vi "Close Hardware.vi"(8 "error in (no error)":errorcluster, 11 "Instrument.VRM in":refnum<class "Instrument.OxfordVRM.lvclass">) -> (0 "error out":errorcluster, 3 "Instrument.VRM out":refnum<class "Instrument.OxfordVRM.lvclass">)   [LabVIEW 2019, in "Instrument.OxfordVRM.lvclass"]
uses:
  Instrument.OxfordVRM.lvclass
  <instrlib>/Mercury iXX/Public/Controls/Mercury Reference.ctl
  <instrlib>/Mercury iXX/Public/Controls/Comms Transport Layer.ctl
  <instrlib>/Mercury iXX/Private/Controls/Query Dynamic Reference.ctl
  Instrument.OxfordVRM.lvclass/Instrument.OxfordVRM.ctl
  <instrlib>/Mercury iXX/Mercury iXX.lvlib
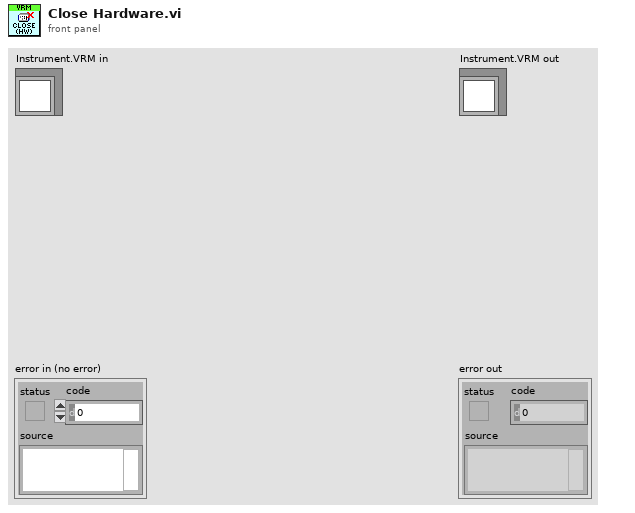
[diagram p1: front panel]
types:
  T1 = typedef "Mercury iXX.lvlib/Mercury Reference.ctl" = cluster{"Comms":refnum<visa-resource-name>, "Device ID":string[], "Comms Layer":T2, "Command":string, "Query reference":T3}
  T2 = typedef "Mercury iXX.lvlib/Comms Transport Layer.ctl" = enum16{"Ethernet TCP/IP", "USB", "ISOBus - RS-232", "GPIB"}
  T3 = typedef "Mercury iXX.lvlib/Query Dynamic Reference.ctl" = refnum<vi>
  T4 = cluster{"Reference":T1, "Devices":cluster{"Temperature":string, "Magnet X":string, "Magnet Y":string, "Magnet Z":string, "PSU 1":string, "PSU 2":string, "PSU 3":string, "PSU 4":string, "PSU 5":string, "PSU 6":string}}
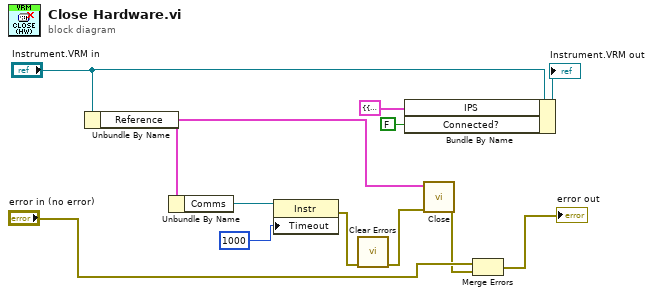
[diagram p0: block diagram]
diagram:
  n1 = Unbundle By Name("Instrument.VRM in") -> ("Reference"=w5:T1)
  n2 = Unbundle By Name(w5) -> ("Comms"=w8:refnum<visa-resource-name>)
  n3 = property class="Instr"(reference=w8, "Timeout"=u32 1000 ("General Settings:Timeout Value")) -> (error out=w6:errorcluster)  [unwired: 1 in, 1 out]
  n4 = call <vilib>:"Clear Errors.vi"("error in (no error)"=w6) -> ("error out"=w4:errorcluster)  [unwired: 5 in, 1 out]
  n5 = Bundle By Name(cluster="Instrument.VRM in", "IPS"=T4 {"Reference"={"Comms"="", "Device ID"=[], "Comms Layer"=enum."Ethernet TCP/IP", "Command"="", "Query reference"=refnum}, "Devices"={"Temperature"="", "Magnet X"="", "Magnet Y"="", "Magnet Z"="", "PSU 1"="", "PSU 2"="", "PSU 3"="", "PSU 4"="", "PSU 5"="", "PSU 6"=""}}, "Connected?"=FALSE ("Connection.Connected?")) -> (→"Instrument.VRM out":refnum<class "Instrument.OxfordVRM.lvclass">)
  n6 = call <instrlib>:"Close.vi"("error in (no error)"=w4, "Mercury Reference"=w5) -> ("error out"=w2:errorcluster)  [unwired: 9 out]
  n7 = Merge Errors("error in (no error)", w2) -> (→"error out":errorcluster)
